vi "data analysis test VI.vi"() -> ()   [LabVIEW 2014]
uses:
  <vilib>/imath/engines/lvmath2/RunTimeEngine/BuiltInFunctions/rand/NIMS_rand(1,I32).vi
  <vilib>/imath/engines/lvmath2/RunTimeEngine/BuiltInFunctions/int16/NIMS_int16(real).vi
  <instcachedir>/0/NIMS_int16(real)_1EFE6F78DFBE4E15B93FF25B3B14BD60.lvgen/NIMS_int16(real)_1EFE6F78DFBE4E15B93FF25B3B14BD60_002.vi
  <vilib>/imath/engines/lvmath2/RunTimeEngine/ErrorHandling/NIMS_Error From Error Code.vi
  <vilib>/imath/engines/lvmath2/RunTimeEngine/BuiltInFunctions/zeros/NIMS_V=zeros(I32,I32).vi
  <vilib>/imath/engines/lvmath2/RunTimeEngine/BuiltInFunctions/int16/NIMS_int16(int).vi
  <instcachedir>/0/NIMS_int16(int)_4445A21B29C14FFE9C78603D13E1117B.lvgen/NIMS_int16(int)_4445A21B29C14FFE9C78603D13E1117B_001.vi
  <vilib>/imathl/engines/lvmath/Functions/Error Handling/Create Error.vi
  <vilib>/imath/engines/lvmath2/RunTimeEngine/RangeToken/NIMS_Range_R2 - Integer.vi
  <instcachedir>/0/NIMS_Range_R2 - Integer_2D1304BAF97744E0A293025746CBADFC.lvgen/NIMS_Range_R2 - Integer_2D1304BAF97744E0A293025746CBADFC_000.vi
  <vilib>/imath/engines/lvmath2/RunTimeEngine/CommandStatement/MC_CommandStatement_break.vi
  <vilib>/imath/engines/lvmath2/RunTimeEngine/IndexRead/NIMS V(S).vi
  <instcachedir>/0/NIMS V(S)_0488751826AF41519A22953C041130DC.lvgen/NIMS V(S)_0488751826AF41519A22953C041130DC_004.vi
  <vilib>/imath/engines/lvmath2/RunTimeEngine/IndexReplace/NIMS V(S)=S.vi
  <instcachedir>/0/NIMS V(S)=S_2D52C4EC15D8415E870AEE69FB516CCA.lvgen/NIMS V(S)=S_2D52C4EC15D8415E870AEE69FB516CCA_003.vi
  <vilib>/imath/engines/lvmath2/RunTimeEngine/ErrorHandling/NIMS_Create Error From Enums.vi
  <instcachedir>/0/NIMS_int16(real)_1EFE6F78DFBE4E15B93FF25B3B14BD60.lvgen/NIMS_int16(real)_1EFE6F78DFBE4E15B93FF25B3B14BD60_000.vi
  <vilib>/imath/engines/lvmath2/RunTimeEngine/NodeEndStatement/NIMS_NodeEndStatement_Output.vi
  <instcachedir>/0/NIMS_NodeEndStatement_Output_53EC0D466D134D7ABD903AC30B43404B.lvgen/NIMS_NodeEndStatement_Output_53EC0D466D134D7ABD903AC30B43404B_012.vi
  <vilib>/imath/engines/lvmath2/RunTimeEngine/ErrorHandling/NIMS_Finalize Error.vi
  <vilib>/imath/engines/lvmath2/RunTimeEngine/BuiltInFunctions/uint16/NIMS_uint16(int).vi
  <instcachedir>/0/NIMS_uint16(int)_AD9B0F7F34DA44259D36ECB142F0DEA3.lvgen/NIMS_uint16(int)_AD9B0F7F34DA44259D36ECB142F0DEA3_001.vi
  <vilib>/imath/engines/lvmath2/RunTimeEngine/IndexReplace/NIMS V(R2)=V.vi
  <instcachedir>/0/NIMS V(R2)=V_680A6DA97A4E4BC09213CA62845C7083.lvgen/NIMS V(R2)=V_680A6DA97A4E4BC09213CA62845C7083_000.vi
  <instcachedir>/0/NIMS_NodeEndStatement_Output_53EC0D466D134D7ABD903AC30B43404B.lvgen/NIMS_NodeEndStatement_Output_53EC0D466D134D7ABD903AC30B43404B_014.vi
panel:
  out "Intensity Graph Y":dbl[][](graph)
  out "Intensity Graph X":dbl[][](graph)
  in  "Scan control":bool
  out "Correlation scanning":bool
  in  "T3 positioning test range (V)":T1
  out "3-1 x correlation":dbl
  out "3-1 y correlation":dbl
  in  "Correlation integration time (s)":dbl
  out "tether forces":waveform(dbl)[](graph)=[{"t0"=timestamp(3.600000000000001 s since 1904-01-01), "dt"=0.1, "Y"=[8.599618085334189, 8.616710768164998], "attributes"=variant("NI_ChannelName"=variant(string "Tether 1"))}, {"t0"=timestamp(3.600000000000001 s since 1904-01-01), "dt"=0.1, "Y"=[8.669934189913317, 8.64500964715035], "attributes"=variant("NI_ChannelName"=variant(string "Tether 2"))}, {"t0"=timestamp(3.600000000000001 s since 1904-01-01), "dt"=0.1, "Y"=[10.029561152841074, 10.043496502647937], "attributes"=variant("NI_ChannelName"=variant(string "Tether 3"))}]
  out "2D tethers":waveform(dbl)[](graph)=[{"t0"=timestamp(3.600000000000001 s since 1904-01-01), "dt"=0.1, "Y"=[930.3826405332136, 929.0101627415797], "attributes"=variant("NI_ChannelName"=variant(string "Tether 1"))}, {"t0"=timestamp(3.600000000000001 s since 1904-01-01), "dt"=0.1, "Y"=[953.5776948104506, 953.7945546499718], "attributes"=variant("NI_ChannelName"=variant(string "Tether 2"))}, {"t0"=timestamp(3.600000000000001 s since 1904-01-01), "dt"=0.1, "Y"=[541.2230047802761, 542.1981030590325], "attributes"=variant("NI_ChannelName"=variant(string "Tether 3"))}]
  in  "Trap 3 Bead Size (nm)":dbl=810.0
  in  "Trap 2 Bead Size (nm)":dbl=810.0
  in  "Trap 1 Bead Size (nm)":dbl=810.0
  out "ratio test":dbl=0.9675233225630537
  in  "Desired forces":T2={"F1x"=7.0, "F1y"=-5.0, "F2x"=-7.0, "F2y"=-5.0}
  in  "Artificial forces":bool=TRUE
  out "Force (pN)":T3={"A_X"=7.0215774989535955, "A_Y"=-4.979745698689579, "B_X"=-7.07501259106649, "B_Y"=-4.989571378686399, "C_X"=-0.031092447141218442, "C_Y"=10.036476588951421}
  out "2D forces":waveform(dbl)[](graph)=[{"t0"=timestamp(3.600000000000001 s since 1904-01-01), "dt"=0.1, "Y"=[7.019682598034811, 7.023472399872379], "attributes"=variant("NI_ChannelName"=variant(string "Trap 1 X"))}, {"t0"=timestamp(3.600000000000001 s since 1904-01-01), "dt"=0.1, "Y"=[-4.967644052914229, -4.991847344464929], "attributes"=variant("NI_ChannelName"=variant(string "Trap 1 Y"))}, {"t0"=timestamp(3.600000000000001 s since 1904-01-01), "dt"=0.1, "Y"=[-7.077163119074762, -7.072862063058218], "attributes"=variant("NI_ChannelName"=variant(string "Trap 2 X"))}, {"t0"=timestamp(3.600000000000001 s since 1904-01-01), "dt"=0.1, "Y"=[-5.008145469476288, -4.97099728789651], "attributes"=variant("NI_ChannelName"=variant(string "Trap 2 Y"))}, {"t0"=timestamp(3.600000000000001 s since 1904-01-01), "dt"=0.1, "Y"=[-0.04011787687321292, -0.022067017409223958], "attributes"=variant("NI_ChannelName"=variant(string "Trap 3 X"))}, {"t0"=timestamp(3.600000000000001 s since 1904-01-01), "dt"=0.1, "Y"=[10.02948091750186, 10.043472260400982], "attributes"=variant("NI_ChannelName"=variant(string "Trap 3 Y"))}]
  in  "Calibration 2":u16(ring)=2 items=["None", "Position", "Force"]
  in  "Calibration":u16(ring)=2 items=["None", "Position", "Force"]
  in  "Displacments":T3={"A_X"=0.0605018, "A_Y"=0.0, "B_X"=0.0507675, "B_Y"=0.0, "C_X"=0.0, "C_Y"=0.0}
  out "Positions \nand displacements":cluster{"X":dbl[], "Y":dbl[]}[](graph)=[{"X"=[3856.9999999999714, 3856.9999999999714], "Y"=[0.0, 0.0]}, {"X"=[6090.0, 6090.0], "Y"=[0.0, 0.0]}, {"X"=[4955.144087038793, 4955.144087038793], "Y"=[-1769.6238715781064, -1769.6238715781064]}, {"X"=[3856.9999999999714, 4191.310570740897, 4191.491059074609], "Y"=[0.0, -233.86603568521076, -235.00547478052496]}, {"X"=[6090.0, 5744.658729782919, 5744.868606554591], "Y"=[0.0, -249.3587186230042, -247.50908725459337]}, {"X"=[4955.144087038793, 4952.707973521867, 4953.804091914954], "Y"=[-1769.6238715781064, -1104.0598883108419, -1103.1314121526243]}, {"X"=[4970.637564152725, 4970.637564152725], "Y"=[-789.6571704971775, -789.6571704971775]}, {"X"=[4952.073488776456, 4952.073488776456], "Y"=[-776.497573056027, -776.497573056027]}, {"X"=[4952.159779557513, 4952.159779557513], "Y"=[-802.6979818639647, -802.6979818639647]}, {"X"=[4958.290277495564, 4958.290277495564], "Y"=[-789.6175751390565, -789.6175751390565]}]
  out "Trap Positions":waveform(dbl)[](graph)=[{"t0"=timestamp(3.600000000000001 s since 1904-01-01), "dt"=0.01, "Y"=[3856.9999999999714, 3856.9999999999714, 3856.9999999999714, 3856.9999999999714, 3856.9999999999714, 3856.9999999999714, 3856.9999999999714, 3856.9999999999714, 3856.9999999999714, 3856.9999999999714, 3856.9999999999714, 3856.9999999999714, 3856.9999999999714, 3856.9999999999714, 3856.9999999999714, 3856.9999999999714, 3856.9999999999714, 3856.9999999999714, 3856.9999999999714, 3856.9999999999714], "attributes"=variant("NI_ChannelName"=variant(string "Trap 1 X"))}, {"t0"=timestamp(3.600000000000001 s since 1904-01-01), "dt"=0.01, "Y"=[6090.0, 6090.0, 6090.0, 6090.0, 6090.0, 6090.0, 6090.0, 6090.0, 6090.0, 6090.0, 6090.0, 6090.0, 6090.0, 6090.0, 6090.0, 6090.0, 6090.0, 6090.0, 6090.0, 6090.0], "attributes"=variant("NI_ChannelName"=variant(string "Trap 2 X"))}, {"t0"=timestamp(3.600000000000001 s since 1904-01-01), "dt"=0.01, "Y"=[4955.144087038793, 4955.144087038793, 4955.144087038793, 4955.144087038793, 4955.144087038793, 4955.144087038793, 4955.144087038793, 4955.144087038793, 4955.144087038793, 4955.144087038793, 4955.144087038793, 4955.144087038793, 4955.144087038793, 4955.144087038793, 4955.144087038793, 4955.144087038793, 4955.144087038793, 4955.144087038793, 4955.144087038793, 4955.144087038793], "attributes"=variant("NI_ChannelName"=variant(string "Trap 3 X"))}, {"t0"=timestamp(3.600000000000001 s since 1904-01-01), "dt"=0.01, "Y"=[-1769.6238715781064, -1769.6238715781064, -1769.6238715781064, -1769.6238715781064, -1769.6238715781064, -1769.6238715781064, -1769.6238715781064, -1769.6238715781064, -1769.6238715781064, -1769.6238715781064, -1769.6238715781064, -1769.6238715781064, -1769.6238715781064, -1769.6238715781064, -1769.6238715781064, -1769.6238715781064, -1769.6238715781064, -1769.6238715781064, -1769.6238715781064, -1769.6238715781064], "attributes"=variant("NI_ChannelName"=variant(string "Trap 3 Y"))}]
  in  "Plot Trap Positions":u16(ring)=1 items=["Relative to Base", "Absolute Positions"]
  in  "Piezo trap y\noffset (V)":dbl=0.6709036530655844
  in  "Piezo trap x\noffset (V)":dbl=-6.361797973205792
  in  "Piezo Trap Y cal (nm/V)":dbl=279.6
  in  "Piezo Trap X cal (nm/V)":dbl=362.7
  in  "AOM X Cal (nm/MHz)":dbl=203.0
  in  "Trap Pos. Disp. Downsample":dbl=1000.0 caption="Trap Downsample"
  in  "Trap 3 Y (V)":dbl=7.0
  in  "Trap 3 X (V)":dbl=7.3
  in  "Trap2 X (MHz)":dbl=90.0
  in  "Trap 1 X (MHz)":dbl=79.0
  in  "Negate Axis":T4={"T1 X"=FALSE, "T2 X"=FALSE, "T3 X"=FALSE, "T3 Y"=TRUE}
  out "Mean":dbl=7.048295045010043 caption="Mean (pN)" format="%#_3g"
  out "T1 X":dbl=7.0215774989535955 caption="T1 X (pN)" format="%0.2f"
  out "T2 X":dbl=7.07501259106649 caption="T2 X (pN)" format="%0.2f"
  out "Difference":dbl=-0.053435092112894544 caption="Difference (pN)" format="%.2g"
  out "Force":waveform(dbl)[](graph)=[{"t0"=timestamp(3.600000000000001 s since 1904-01-01), "dt"=0.1, "Y"=[7.019682598034811, 7.023472399872379], "attributes"=variant("NI_ChannelName"=variant(string "Trap 1 X"))}, {"t0"=timestamp(3.600000000000001 s since 1904-01-01), "dt"=0.1, "Y"=[7.077163119074762, 7.072862063058218], "attributes"=variant("NI_ChannelName"=variant(string "Trap 2 X"))}, {"t0"=timestamp(3.600000000000001 s since 1904-01-01), "dt"=0.1, "Y"=[7.048422858554787, 7.048167231465298], "attributes"=variant("NI_ChannelName"=variant(string "Mean"))}]
  in  "Mean Trap Positions (nm)":T5={"T1 X"=3856.9999999999714, "T2 X"=6090.0, "T3 X"=4955.144087038793, "T3 Y"=-1769.6238715781064} {"T3 Y" format="%#_6f"; "T3 X" format="%#_6f"; "T2 X" format="%#_6f"; "T1 X" format="%#_6f"}
  in  "Path":path=path "C:/Data/180321/current.off"
  in  "Read Cal":bool
  out "Read cal error":errorcluster
  in  "T3 calibration":T6={"alpha_x (nm/V)"=705.7585317734071, "offset_x (mV)"=-72.05792299729328, "kappa_x (pN/nm)"=0.32935966730993543, "alpha_y (nm/V)"=745.2903215958727, "kappa_y (pN/nm)"=0.3013829224432179, "offset_y (mV)"=22.362021368510735} {"offset_y (mV)" format="%#_2g"; "kappa_y (pN/nm)" min=0.0 step=0.001 format="%#_2g"; "alpha_y (nm/V)" step=10.0 format="%#_3g"; "kappa_x (pN/nm)" min=0.0 step=0.001 format="%#_2g"; "offset_x (mV)" format="%#_2g"; "alpha_x (nm/V)" step=10.0 format="%#_3g"}
  in  "T2 calibration":T6={"alpha_x (nm/V)"=564.800175494257, "offset_x (mV)"=-41.69276077209905, "kappa_x (pN/nm)"=0.40986489188657144, "alpha_y (nm/V)"=679.2654766858733, "kappa_y (pN/nm)"=0.40168200230832185, "offset_y (mV)"=-0.41558808755755094} {"offset_y (mV)" format="%#_2g"; "kappa_y (pN/nm)" min=0.0 step=0.001 format="%#_2g"; "alpha_y (nm/V)" step=10.0 format="%#_3g"; "kappa_x (pN/nm)" min=0.0 step=0.001 format="%#_2g"; "offset_x (mV)" format="%#_2g"; "alpha_x (nm/V)" step=10.0 format="%#_3g"}
  in  "T1 calibration":T6={"alpha_x (nm/V)"=544.9680094639928, "offset_x (mV)"=-33.70790453197266, "kappa_x (pN/nm)"=0.4199497839674786, "alpha_y (nm/V)"=662.8467814087468, "kappa_y (pN/nm)"=0.424828174673538, "offset_y (mV)"=32.28801513873096} {"offset_y (mV)" format="%#_2g"; "kappa_y (pN/nm)" min=0.0 step=0.001 format="%#_2g"; "alpha_y (nm/V)" step=10.0 format="%#_3g"; "kappa_x (pN/nm)" min=0.0 step=0.001 format="%#_2g"; "offset_x (mV)" format="%#_2g"; "alpha_x (nm/V)" step=10.0 format="%#_3g"}
  in  "Multi-MCL offset array":T7(array[cluster])
  in  "Two Trap Offset Values":T8={"Trap 1X offset"=array[1799 elements], "Trap 2X offset"=array[1799 elements]}
  in  "MCL offset scanning range (V)":T9={"Min X"=6.0, "Max X"=9.0, "Min Y"=5.0, "Max Y"=8.0, "Scan increment"=1.0}
  in  "Dynamic offset\nupdate":bool=TRUE
  in  "Offset file step size":dbl=0.1
  out "Array":i16[](array[numeric])
  in  "stop":bool
  in  "Multiple-MCL offset?":bool=TRUE
  in  "DMA period (s)":dbl=0.2
  in  "dataperiod (us)":dbl=10.0
  in  "trap sets":u32=2
  in  "Flip X Sign":bool
  in  "Detector Type":string(combo)="IR-QPD + PSD + FB-QPD X position"
  in  "Trap Disp. Downsample":dbl=10000.0 caption="Downsample" max=20000.0
  out "All Signals":waveform(dbl)[](graph)=[{"t0"=timestamp(3.600000000000001 s since 1904-01-01), "dt"=0.1, "Y"=[0.0008898377716559546, 0.000803887358432814], "attributes"=variant("NI_ChannelName"=variant(string "T1 Y"))}, {"t0"=timestamp(3.600000000000001 s since 1904-01-01), "dt"=0.1, "Y"=[-0.004640863177226808, -0.00462430364248546], "attributes"=variant("NI_ChannelName"=variant(string "T1 X"))}, {"t0"=timestamp(3.600000000000001 s since 1904-01-01), "dt"=0.1, "Y"=[0.997039704580851, 0.997039704580851], "attributes"=variant("NI_ChannelName"=variant(string "T1 Sum"))}, {"t0"=timestamp(3.600000000000001 s since 1904-01-01), "dt"=0.1, "Y"=[-0.01875053565962656, -0.018614386287113534], "attributes"=variant("NI_ChannelName"=variant(string "T2 Y"))}, {"t0"=timestamp(3.600000000000001 s since 1904-01-01), "dt"=0.1, "Y"=[-0.07344958677685948, -0.07343100704009785], "attributes"=variant("NI_ChannelName"=variant(string "T2 X"))}, {"t0"=timestamp(3.600000000000001 s since 1904-01-01), "dt"=0.1, "Y"=[0.997039704580851, 0.997039704580851], "attributes"=variant("NI_ChannelName"=variant(string "T2 Sum"))}, {"t0"=timestamp(3.600000000000001 s since 1904-01-01), "dt"=0.1, "Y"=[-2.8313437404346336e-05, -2.907866544230067e-06], "attributes"=variant("NI_ChannelName"=variant(string "T1 FB X"))}, {"t0"=timestamp(3.600000000000001 s since 1904-01-01), "dt"=0.1, "Y"=[0.997039704580851, 0.997039704580851], "attributes"=variant("NI_ChannelName"=variant(string "T1 FB Sum"))}, {"t0"=timestamp(3.600000000000001 s since 1904-01-01), "dt"=0.1, "Y"=[-2.684419957147232e-05, 1.8702173247627797e-05], "attributes"=variant("NI_ChannelName"=variant(string "T2 FB X"))}, {"t0"=timestamp(3.600000000000001 s since 1904-01-01), "dt"=0.1, "Y"=[0.997039704580851, 0.997039704580851], "attributes"=variant("NI_ChannelName"=variant(string "T2 FB Sum"))}, {"t0"=timestamp(3.600000000000001 s since 1904-01-01), "dt"=0.1, "Y"=[0.06976369758187939, 0.06982598714416899], "attributes"=variant("NI_ChannelName"=variant(string "T3 Y/ PSD Y"))}, {"t0"=timestamp(3.600000000000001 s since 1904-01-01), "dt"=0.1, "Y"=[-0.07324104683195597, -0.07316339149066425], "attributes"=variant("NI_ChannelName"=variant(string "T3 X / PSD X"))}, {"t0"=timestamp(3.600000000000001 s since 1904-01-01), "dt"=0.1, "Y"=[0.997039704580851, 0.997039704580851], "attributes"=variant("NI_ChannelName"=variant(string "T3 Sum / PSD sum"))}]
  # "1 D forces traps 1 and 2"
  # "2D forces"
  # "2D tethers"
  # "Individual tether forces"
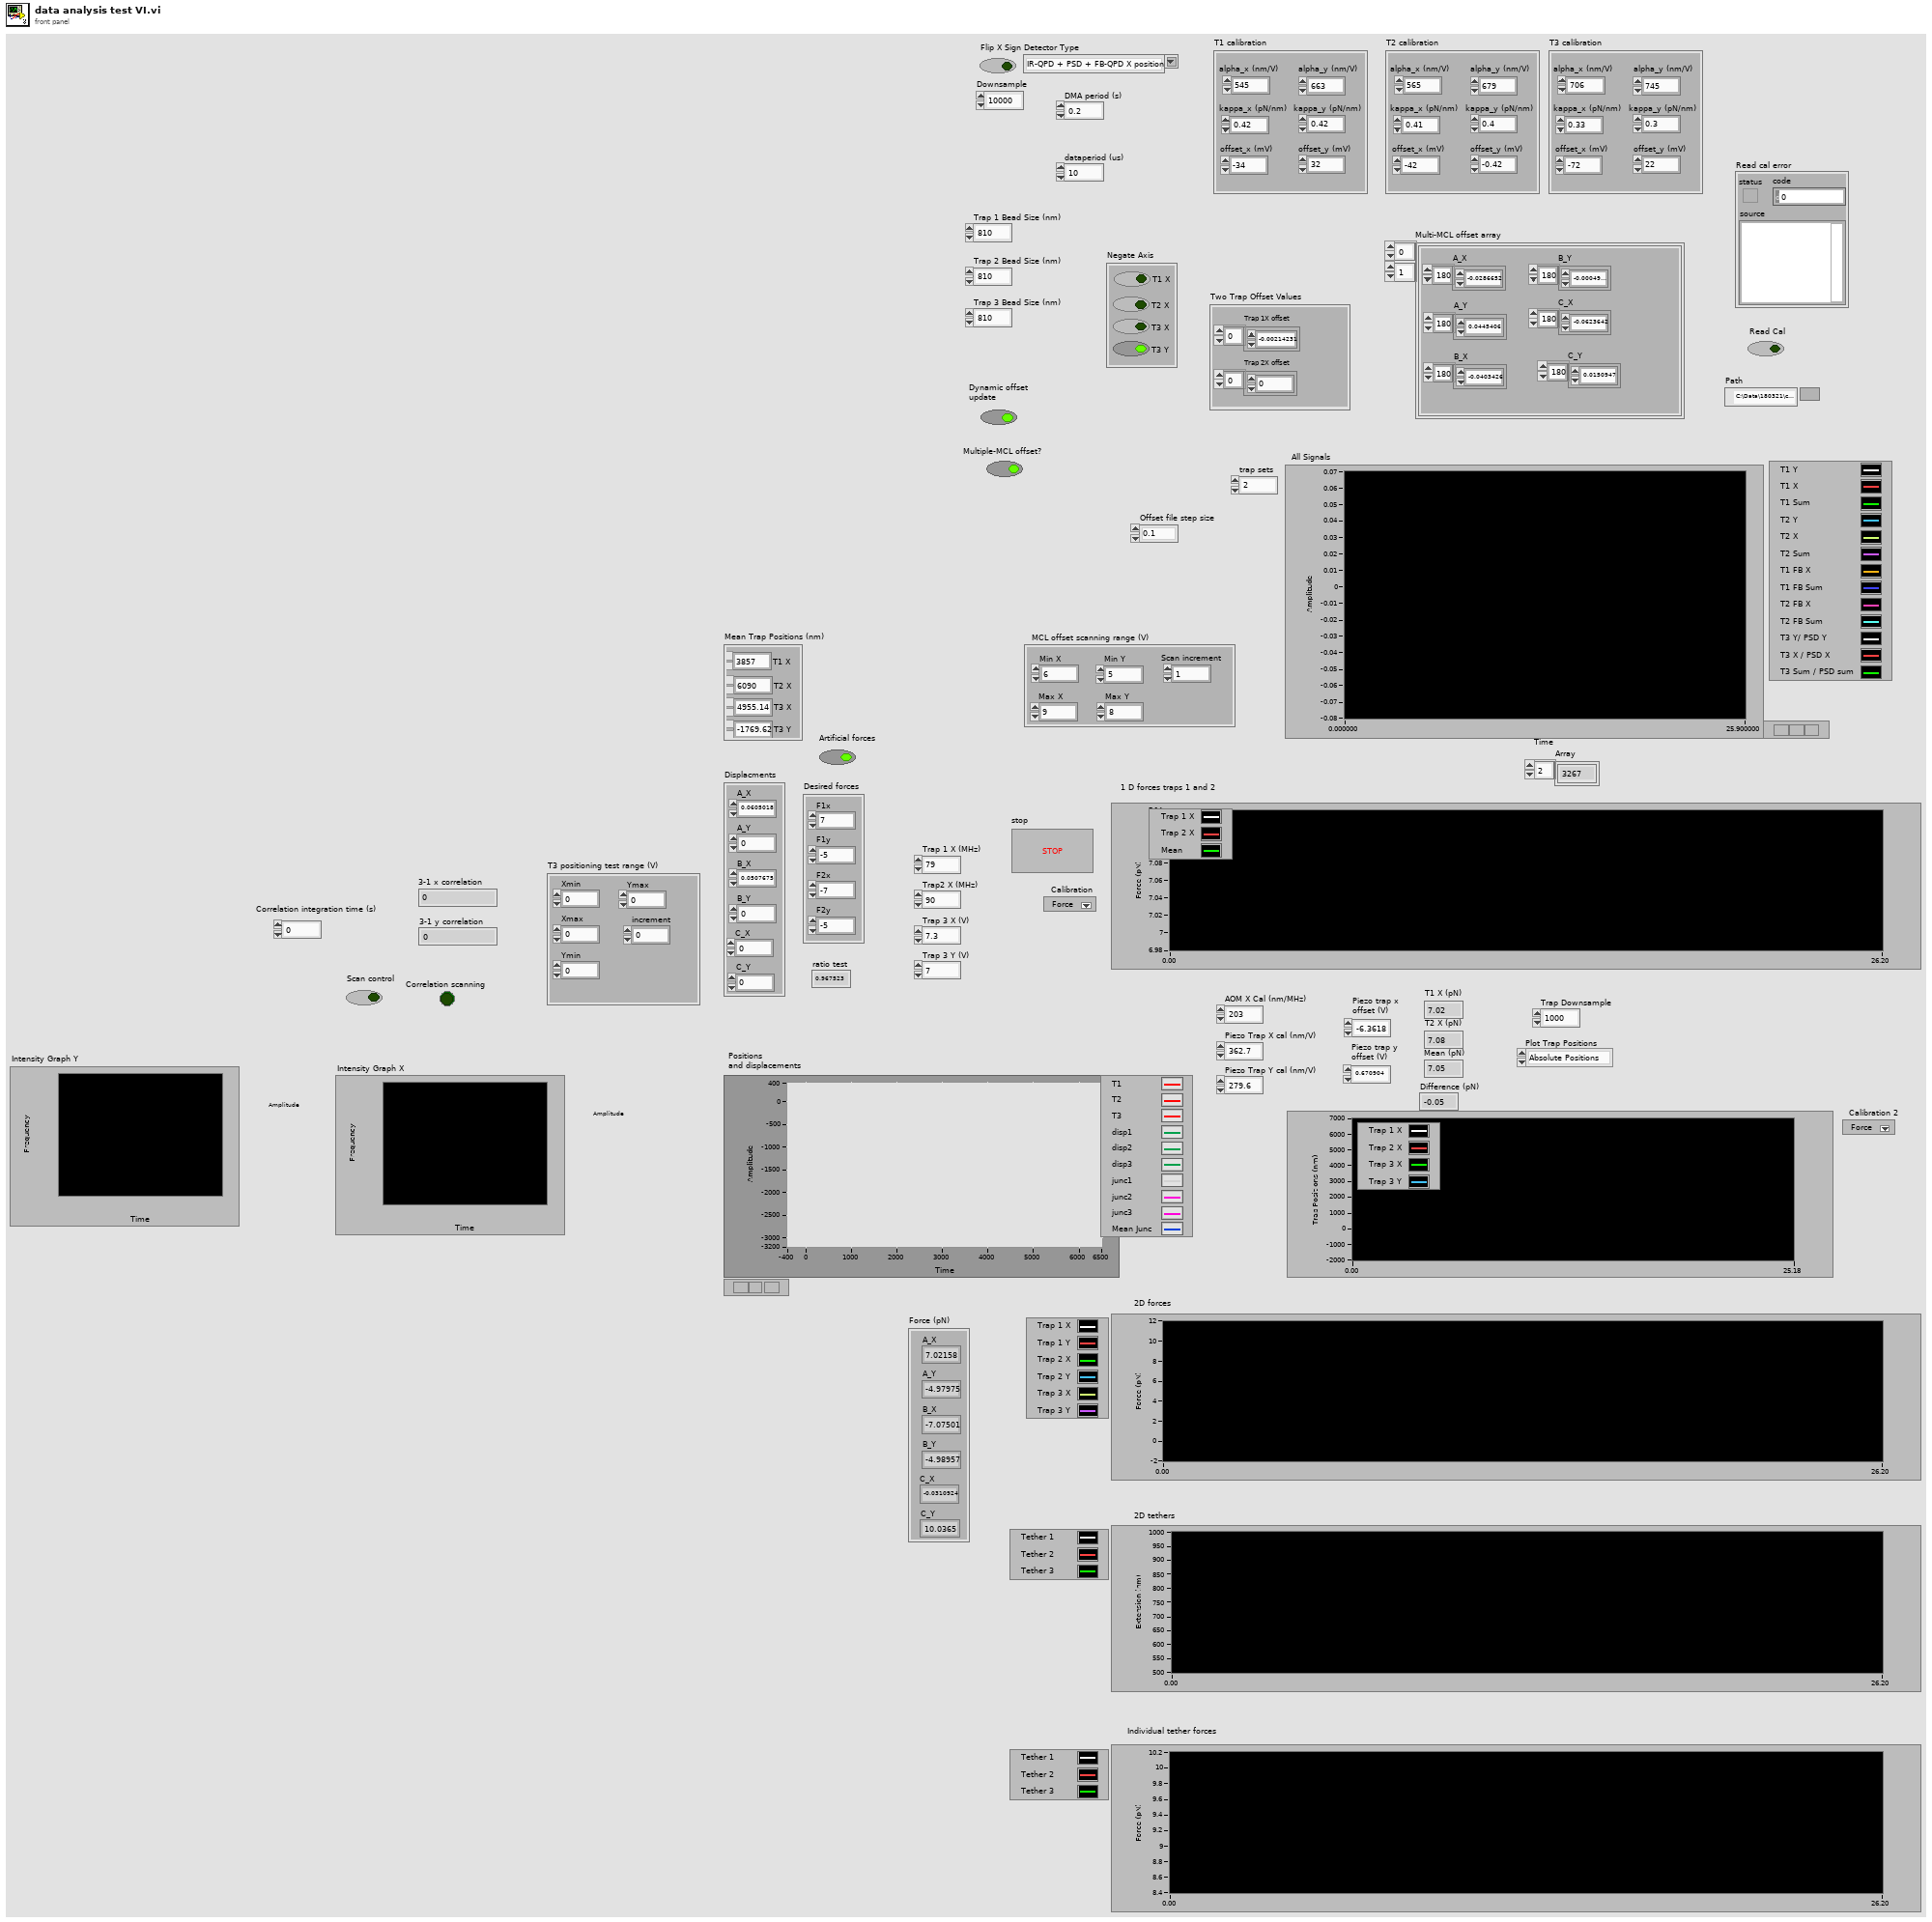
[diagram p1: front panel]
types:
  T1 = cluster{"Xmin":dbl, "Xmax":dbl, "Ymin":dbl, "Ymax":dbl, "increment":dbl}
  T2 = cluster{"F1x":dbl, "F1y":dbl, "F2x":dbl, "F2y":dbl}
  T3 = cluster{"A_X":dbl, "A_Y":dbl, "B_X":dbl, "B_Y":dbl, "C_X":dbl, "C_Y":dbl}
  T4 = cluster{"T1 X":bool, "T2 X":bool, "T3 X":bool, "T3 Y":bool}
  T5 = cluster{"T1 X":dbl, "T2 X":dbl, "T3 X":dbl, "T3 Y":dbl}
  T6 = cluster{"alpha_x (nm/V)":dbl, "offset_x (mV)":dbl, "kappa_x (pN/nm)":dbl, "alpha_y (nm/V)":dbl, "kappa_y (pN/nm)":dbl, "offset_y (mV)":dbl}
  T7 = cluster{"A_X":dbl[], "A_Y":dbl[], "B_X":dbl[], "B_Y":dbl[], "C_X":dbl[], "C_Y":dbl[]}[][]
  T8 = cluster{"Trap 1X offset":dbl[], "Trap 2X offset":dbl[]}
  T9 = cluster{"Min X":dbl, "Max X":dbl, "Min Y":dbl, "Max Y":dbl, "Scan increment":dbl}
  T10 = enum16{"open", "replace", "create", "open or create", "replace or create", "replace or create with confirmation"}
  T11 = enum16{"big-endian, network order", "native, host order", "little-endian"}
  T12 = cluster{"alpha_x (nm/V)":dbl, "offset_x (mV)":dbl, "kappa_x (pN/nm)":dbl, "alpha_y (nm/V)":dbl, "kappa_y (pN/nm)":dbl, "offset_y (mV)":dbl}[]
  T13 = cluster{"[0]":dbl, "[1]":dbl, "[2]":dbl, "[3]":dbl, "[4]":dbl, "[5]":dbl}
  T14 = cluster{"Output trap positions[0]":cluster{"X":dbl[], "Y":dbl[]}, "Output trap positions[1]":cluster{"X":dbl[], "Y":dbl[]}, "Output trap positions[2]":cluster{"X":dbl[], "Y":dbl[]}}
  T15 = cluster{"X correlation":dbl, "Y correlation":dbl}
  T16 = cluster{"T1 X":dbl, "T2 X":dbl, "Mean":dbl, "Difference":dbl}
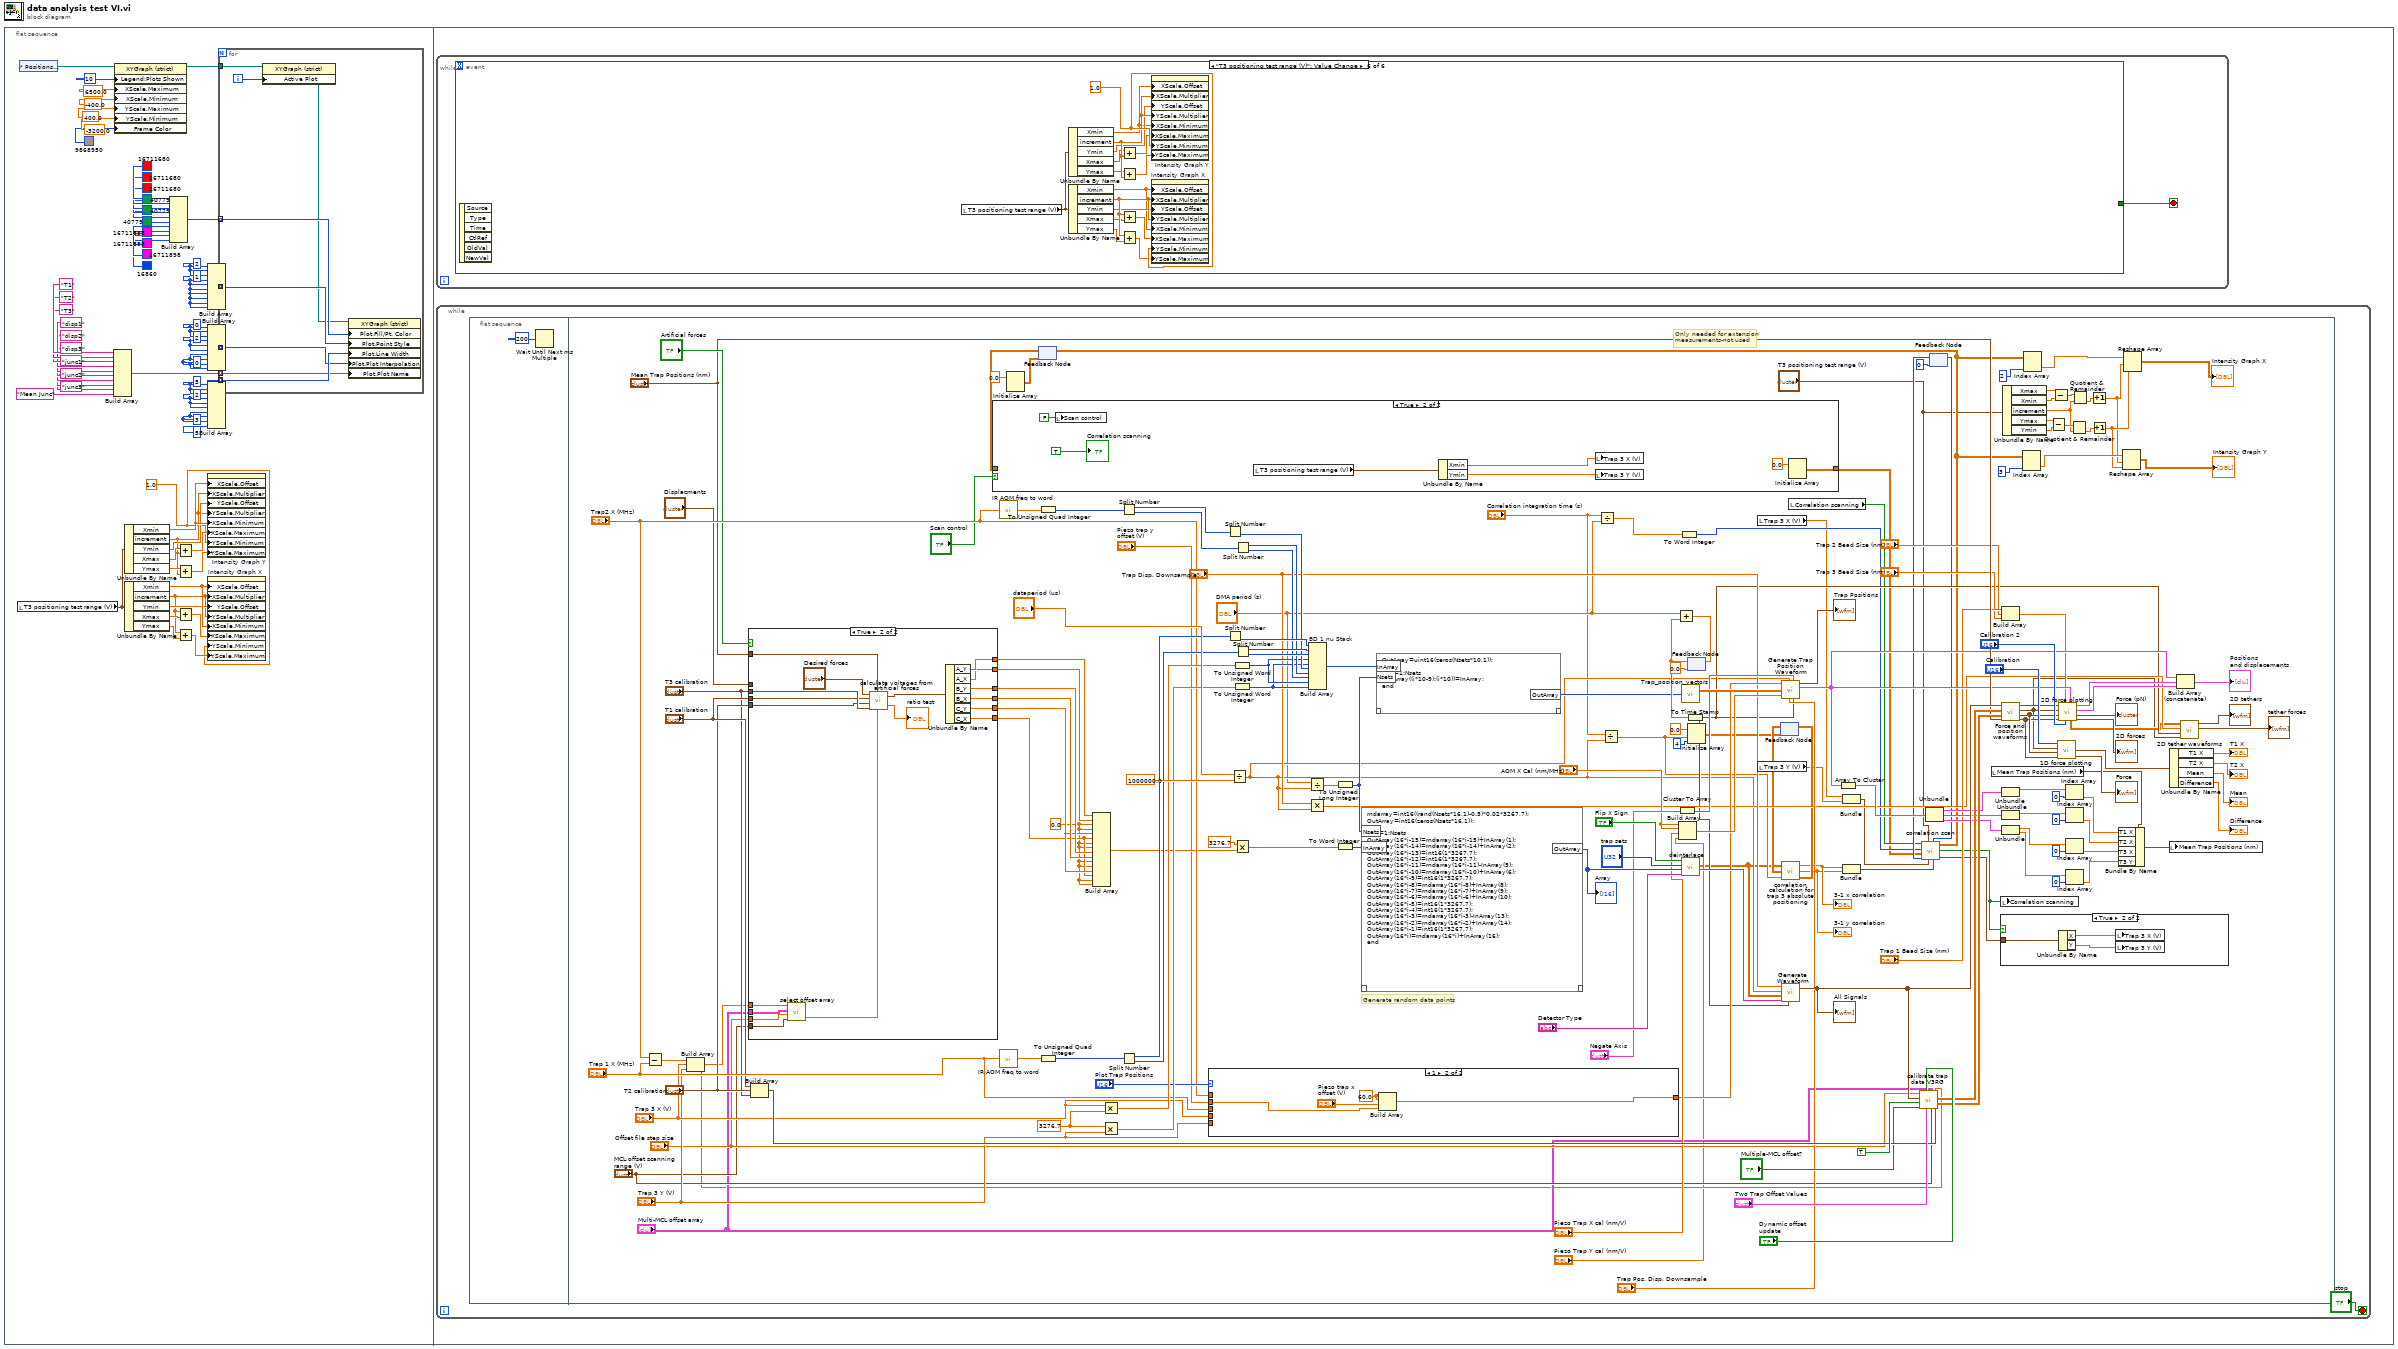
[diagram p0: block diagram]
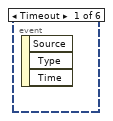
[diagram p2: hidden frame]
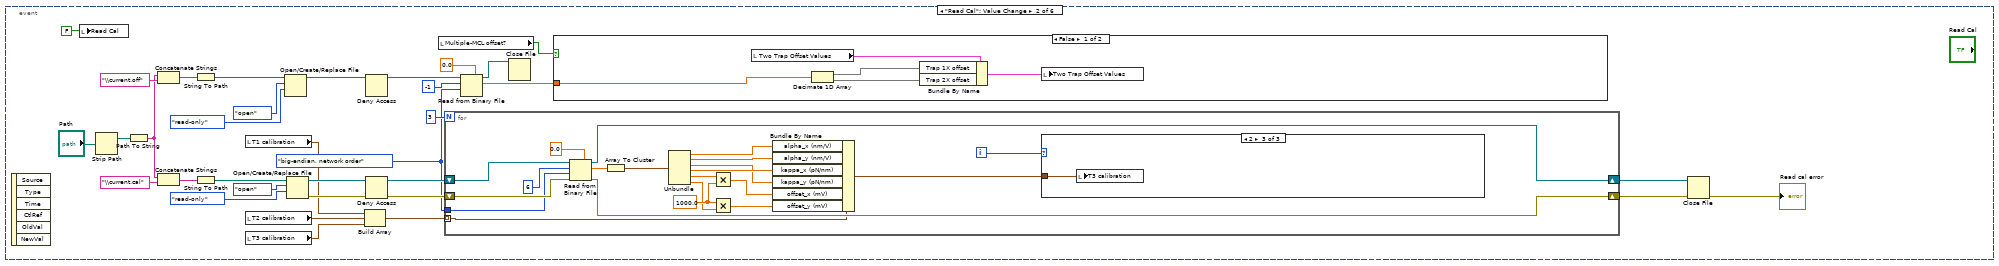
[diagram p3: hidden frame]
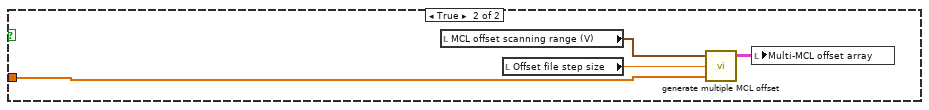
[diagram p4: hidden frame]
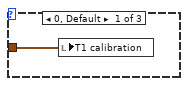
[diagram p5: hidden frame]
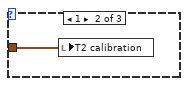
[diagram p6: hidden frame]
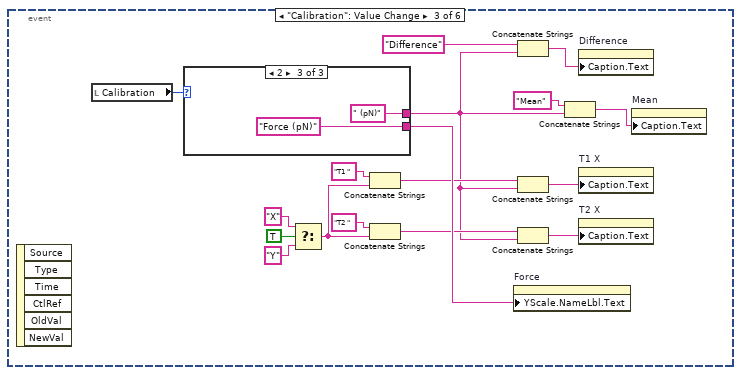
[diagram p7: hidden frame]
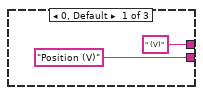
[diagram p8: hidden frame]
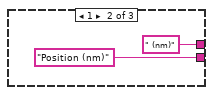
[diagram p9: hidden frame]
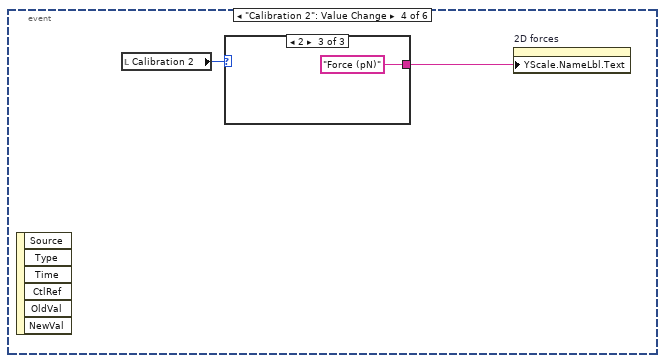
[diagram p10: hidden frame]
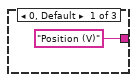
[diagram p11: hidden frame]
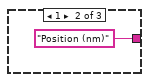
[diagram p12: hidden frame]
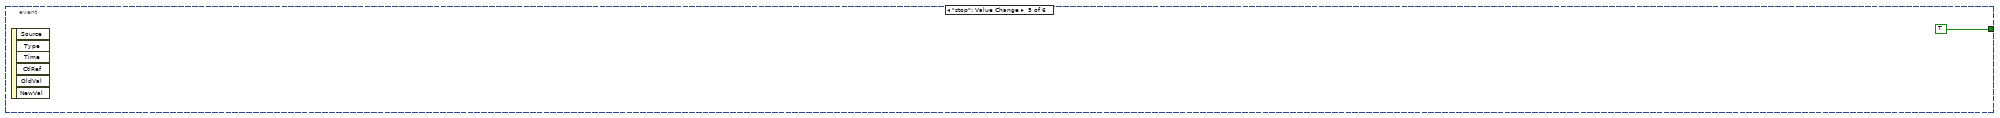
[diagram p13: hidden frame]
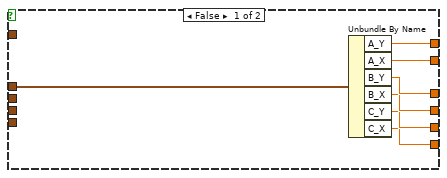
[diagram p16: hidden frame]
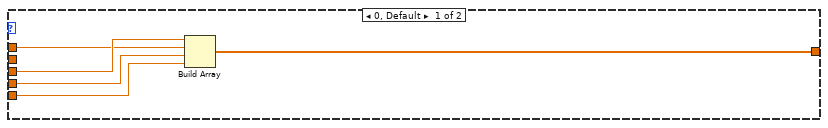
[diagram p17: hidden frame]
diagram:
  n1 = flat-sequence {
    frame #0 {
      w1 = 1.0
      w29 = 0
      w30 = 2
      w31 = 0
      w34 = 3
      w35 = 2
      w36 = 5
      w38 = 1
      w39 = 2
      n2 = local read "T3 positioning test range (V)"() -> (w16:T1)
      n3 = control-ref of="Positions \nand displacements"() -> (w58:refnum<vi>)
      n4 = Build Array("T1", "T2", "T3", "disp1", "disp2", "disp3", "junc1", "junc2", "junc3", "Mean Junc") -> (w17:string[])
      n5 = property class="XYGraph (strict)"(reference=w58, "Legend:Plots Shown"=10, "XScale.Maximum"=6500.0, "XScale.Minimum"=-400.0, "YScale.Maximum"=400.0, "YScale.Minimum"=-3200.0, "Frame Color"=u32 9868950) -> (reference out=w51:refnum<vi>)  [unwired: 1 in, 1 out]
      n6 = Unbundle By Name(w16) -> ("Xmin"=w15:dbl, "increment"=w10:dbl, "Ymin"=w12:dbl, "Xmax"=w14:dbl, "Ymax"=w11:dbl)
      n7 = Unbundle By Name(w16) -> ("Xmin"=w8:dbl, "increment"=w3:dbl, "Ymin"=w7:dbl, "Xmax"=w6:dbl, "Ymax"=w4:dbl)
      n8 = Build Array(u32 16711680, u32 16711680, u32 16711680, u32 40779, u32 40779, u32 40779, u32 16711898, u32 16711898, u32 16711898, u32 16860) -> (w40:u32[])
      n9 = Add(x=w14, y=w10) -> (x+y=w13:dbl)
      n10 = Add(x=w11, y=w10) -> (x+y=w9:dbl)
      n11 = Add(x=w3, y=w6) -> (x+y=w5:dbl)
      n12 = Add(x=w3, y=w4) -> (x+y=w2:dbl)
      n13 = Build Array(w39, w39, w39, w38, w38, w38, w38, w38, w38, w38) -> (w37:i32[])
      n14 = Build Array(w31, w31, w31, w30, w30, w30, w29, w29, w29, w29) -> (w28:i32[])
      n15 = Build Array(w36, w36, w36, w35, w35, w35, w34, w34, w34, 5) -> (w32:i32[])
      n16 = property on="Intensity Graph Y" class="IntGraph (strict)"("XScale.Offset"=w15, "XScale.Multiplier"=w10, "YScale.Offset"=w12, "YScale.Multiplier"=w10, "XScale.Minimum"=w15, "XScale.Maximum"=w13, "YScale.Minimum"=w1, "YScale.Maximum"=w9) -> ()  [unwired: 2 in, 2 out]
      n17 = property on="Intensity Graph X" class="IntGraph (strict)"("XScale.Offset"=w8, "XScale.Multiplier"=w3, "YScale.Offset"=w7, "YScale.Multiplier"=w3, "XScale.Minimum"=w8, "XScale.Maximum"=w5, "YScale.Minimum"=w1, "YScale.Maximum"=w2) -> ()  [unwired: 2 in, 2 out]
      n18 = for {
        tunnel: w51 -> [w66]
        tunnel: w40 -> [w64] mode=indexing
        tunnel: w37 -> [w63] mode=indexing
        tunnel: w32 -> [w62] mode=indexing
        tunnel: w28 -> [w61] mode=indexing
        tunnel: w17 -> [w59] mode=indexing
        i -> [w65]
        n19 = property class="XYGraph (strict)"(reference=w66, "Active Plot"=w65) -> (reference out=w60:refnum<vi>)  [unwired: 1 in, 1 out]
        n20 = property class="XYGraph (strict)"(reference=w60, "Plot.Fill/Pt. Color"=w64, "Plot.Point Style"=w63, "Plot.Line Width"=w62, "Plot.Plot Interpolation"=w61, "Plot.Plot Name"=w59) -> ()  [unwired: 1 in, 2 out]
      }
    }
    frame #1 {
      n21 = while {
        stop <- w67 stop-if-true
        n22 = event shown="[5] \"T3 positioning test range (V)\": Value Change" {
          selector: _ -> [_ _ _ _ _ _]
          dyn-events: _ -> [_ _ _ _ _ _]
          timeout: _ -> [_ _ _ _ _ _]
          tunnel: [_ _ _ _ TRUE _] -> w67
          event Timeout {
            n23 = event-data() -> ()  [unwired: 1 in, 3 out]
          }
          event "Read Cal": Value Change {
            w79 = T11."big-endian, network order" ("byte order (0:big-endian, network order)")
            n24 = event-data() -> ()  [unwired: 1 in, 6 out]
            n25 = local write "Read Cal"(FALSE) -> ()
            n26 = Strip Path(path="Path") -> (stripped path=w88:path)  [unwired: 1 out]
            n27 = Path To String(path=w88) -> (string=w93:string)
            n28 = Concatenate Strings(w93, "\\current.off" ("string")) -> (w95:string)
            n29 = Concatenate Strings(w93, "\\current.cal" ("string")) -> (w90:string)
            n30 = String To Path(string=w95) -> (path=w98:path)
            n31 = String To Path(string=w90) -> (path=w91:path)
            n32 = local read "T1 calibration"() -> (w78:T6)
            n33 = local read "T2 calibration"() -> (w77:T6)
            n34 = local read "T3 calibration"() -> (w76:T6)
            n35 = Open/Create/Replace File(file path (use dialog)=w98, operation (0:open)=T10."open", access (0:read/write)=enum16{"read/write", "read-only", "write-only"}."read-only") -> (refnum out=w99:refnum<file>)  [unwired: 1 in, 4 out]
            n36 = Open/Create/Replace File(file path (use dialog)=w91, operation (0:open)=T10."open", access (0:read/write)=enum16{"read/write", "read-only", "write-only"}."read-only") -> (refnum out=w85:refnum<file>, error out=w92:errorcluster)  [unwired: 1 in, 3 out]
            n37 = Build Array(w78, w77, w76) -> (w75:T12)
            n38 = Deny Access(7:w99) -> (3:w100:refnum<file>)  [unwired: 1 in, 2 out]
            n39 = Deny Access(4:w92, 7:w85) -> (0:w80:errorcluster, 3:w81:refnum<file>)  [unwired: 1 out]
            n40 = local read "Multiple-MCL offset?"() -> (w73:bool)
            n41 = for {
              N: 3 -> [_]
              shift-right: [w117] -> w70
              shift-left: w81 -> [w118]
              shift-right: [w115] -> w69
              shift-left: w80 -> [w116]
              tunnel: w79 -> [w114]
              tunnel: w75 -> [w113] mode=indexing
              i -> [w112]
              w130 = 1000.0
              n42 = Read from Binary File(5:0.0, 8:w116, 9:w114, 10:6 ("count (1)"), 11:w118) -> (0:w115:errorcluster, 2:w119:dbl[], 3:w117:refnum<file>)  [unwired: 2 out]
              n43 = Array To Cluster(array=w119) -> (cluster=w122:T13)
              n44 = Unbundle(w122) -> ("[0]"=w123:dbl, "[1]"=w124:dbl, "[2]"=w128:dbl, "[3]"=w125:dbl, "[4]"=w129:dbl, "[5]"=w126:dbl)
              n45 = Multiply(x=w129, y=w130) -> (x*y=w131:dbl)
              n46 = Multiply(x=w130, y=w126) -> (x*y=w127:dbl)
              n47 = Bundle By Name(cluster=w113, "alpha_x (nm/V)"=w123, "alpha_y (nm/V)"=w124, "kappa_x (pN/nm)"=w128, "kappa_y (pN/nm)"=w125, "offset_x (mV)"=w131, "offset_y (mV)"=w127) -> (w111:T6)
              n48 = case shown="2" w112 {
                tunnel: w111 -> [w132 w133 w134]
                frame 0, Default {
                  n49 = local write "T1 calibration"(w132) -> ()
                }
                frame 1 {
                  n50 = local write "T2 calibration"(w133) -> ()
                }
                frame 2 {
                  n51 = local write "T3 calibration"(w134) -> ()
                }
              }
            }
            n52 = Read from Binary File(5:0.0, 9:w79, 10:-1 ("count (1)"), 11:w100) -> (2:w72:dbl[], 3:w83:refnum<file>)  [unwired: 1 in, 3 out]
            n53 = Close File(refnum=w83) -> ()  [unwired: 1 in, 2 out]
            n54 = case shown="False" w73 {
              tunnel: w72 -> [w106 w108]
              frame False {
                n55 = local read "Two Trap Offset Values"() -> (w105:T8)
                n56 = Decimate 1D Array(w106) -> (w104:dbl[], w103:dbl[])
                n57 = Bundle By Name(cluster=w105, "Trap 1X offset"=w104, "Trap 2X offset"=w103) -> (w102:T8)
                n58 = local write "Two Trap Offset Values"(w102) -> ()
              }
              frame True {
                n59 = local read "MCL offset scanning range (V)"() -> (w110:T9)
                n60 = local read "Offset file step size"() -> (w109:dbl)
                n61 = call "generate multiple MCL offset.vi"("Offset array"=w108, "offset file step size"=w109, "MCL offset scanning range (V)"=w110) -> ("Output array"=w107:T7)  [unwired: 2 out]
                n62 = local write "Multi-MCL offset array"(w107) -> ()
              }
            }
            n63 = Close File(refnum=w70, error in=w69) -> (error out=→"Read cal error":errorcluster)  [unwired: 1 out]
          }
          event "Calibration": Value Change {
            n64 = event-data() -> ()  [unwired: 1 in, 6 out]
            n65 = local read "Calibration"() -> (w151:u16)
            n66 = case shown="2" w151 {
              tunnel: ["Position (V)" ("Label.Text") "Position (nm)" ("Label.Text") "Force (pN)" ("Label.Text")] -> w150
              tunnel: [" (V)" ("Label.Text") " (nm)" ("Label.Text") " (pN)" ("Label.Text")] -> w139
              frame 0, Default {
              }
              frame 1 {
              }
              frame 2 {
              }
            }
            n67 = Select(t="X" ("Label.Text"), s=TRUE, f="Y" ("Label.Text")) -> (s? t:f=w144:string)
            n68 = Concatenate Strings("T1 " ("Label.Text"), w144) -> (w147:string)
            n69 = Concatenate Strings("T2 " ("Label.Text"), w144) -> (w148:string)
            n70 = property on="Force" class="WFChart (strict)"("YScale.NameLbl.Text"=w150) -> ()  [unwired: 2 in, 2 out]
            n71 = Concatenate Strings("Difference" ("Label.Text"), w139) -> (w135:string)
            n72 = Concatenate Strings(w147, w139) -> (w137:string)
            n73 = Concatenate Strings(w148, w139) -> (w136:string)
            n74 = Concatenate Strings("Mean" ("Label.Text"), w139) -> (w138:string)
            n75 = property on="Difference" class="DigNum (strict)"("Caption.Text"=w135) -> ()  [unwired: 2 in, 2 out]
            n76 = property on="T1 X" class="DigNum (strict)"("Caption.Text"=w137) -> ()  [unwired: 2 in, 2 out]
            n77 = property on="T2 X" class="DigNum (strict)"("Caption.Text"=w136) -> ()  [unwired: 2 in, 2 out]
            n78 = property on="Mean" class="DigNum (strict)"("Caption.Text"=w138) -> ()  [unwired: 2 in, 2 out]
          }
          event "Calibration 2": Value Change {
            n79 = event-data() -> ()  [unwired: 1 in, 6 out]
            n80 = local read "Calibration 2"() -> (w159:u16)
            n81 = case shown="2" w159 {
              tunnel: ["Position (V)" ("Label.Text") "Position (nm)" ("Label.Text") "Force (pN)" ("Label.Text")] -> w158
              frame 0, Default {
              }
              frame 1 {
              }
              frame 2 {
              }
            }
            n82 = property on="2D forces" class="WFChart (strict)"("YScale.NameLbl.Text"=w158) -> ()  [unwired: 2 in, 2 out]
          }
          event "stop": Value Change {
            n83 = event-data() -> ()  [unwired: 1 in, 6 out]
          }
          event "T3 positioning test range (V)": Value Change {
            w179 = 1.0
            n84 = event-data() -> ()  [unwired: 1 in, 6 out]
            n85 = local read "T3 positioning test range (V)"() -> (w164:T1)
            n86 = Unbundle By Name(w164) -> ("Xmin"=w165:dbl, "increment"=w170:dbl, "Ymin"=w168:dbl, "Xmax"=w166:dbl, "Ymax"=w169:dbl)
            n87 = Unbundle By Name(w164) -> ("Xmin"=w172:dbl, "increment"=w177:dbl, "Ymin"=w173:dbl, "Xmax"=w174:dbl, "Ymax"=w176:dbl)
            n88 = Add(x=w166, y=w170) -> (x+y=w167:dbl)
            n89 = Add(x=w169, y=w170) -> (x+y=w171:dbl)
            n90 = Add(x=w177, y=w174) -> (x+y=w175:dbl)
            n91 = Add(x=w177, y=w176) -> (x+y=w178:dbl)
            n92 = property on="Intensity Graph Y" class="IntGraph (strict)"("XScale.Offset"=w165, "XScale.Multiplier"=w170, "YScale.Offset"=w168, "YScale.Multiplier"=w170, "XScale.Minimum"=w165, "XScale.Maximum"=w167, "YScale.Minimum"=w179, "YScale.Maximum"=w171) -> ()  [unwired: 2 in, 2 out]
            n93 = property on="Intensity Graph X" class="IntGraph (strict)"("XScale.Offset"=w172, "XScale.Multiplier"=w177, "YScale.Offset"=w173, "YScale.Multiplier"=w177, "XScale.Minimum"=w172, "XScale.Maximum"=w175, "YScale.Minimum"=w179, "YScale.Maximum"=w178) -> ()  [unwired: 2 in, 2 out]
          }
        }
      }
      n94 = while {
        stop <- "stop" stop-if-true
        n95 = flat-sequence {
          frame #0 {
            n96 = Wait Until Next ms Multiple(millisecond multiple=u32 200) -> ()  [unwired: 1 out]
          }
          frame #1 {
            w286 = 0.0
            w313 = 3276.7
            # "Only needed for extension\nmeasurements-not used"
            # "Generate random data points"
            n97 = Subtract(x="Trap2 X (MHz)", y="Trap 1 X (MHz)") -> (x-y=w296:dbl)
            n98 = Build Array(w296, "Trap 3 X (V)", "Trap 3 Y (V)") -> (w265:dbl[])
            n99 = case shown="True" "Artificial forces" {
              tunnel: "Displacments" -> [w372 _]
              tunnel: [w371 w388] -> w292
              tunnel: [w370 w387] -> w291
              tunnel: [w369 w386] -> w290
              tunnel: [w368 w384] -> w289
              tunnel: [w367 w383] -> w288
              tunnel: [w366 w385] -> w287
              tunnel: "T1 calibration" -> [_ w381]
              tunnel: "T2 calibration" -> [_ w380]
              tunnel: "T3 calibration" -> [_ w382]
              tunnel: "Mean Trap Positions (nm)" -> [_ w374]
              tunnel: "Offset file step size" -> [_ w379]
              tunnel: "MCL offset scanning range (V)" -> [_ w378]
              tunnel: "Multi-MCL offset array" -> [_ w377]
              tunnel: w265 -> [_ w376]
              frame False {
                n100 = Unbundle By Name(w372) -> ("A_Y"=w371:dbl, "A_X"=w370:dbl, "B_Y"=w369:dbl, "B_X"=w368:dbl, "C_Y"=w367:dbl, "C_X"=w366:dbl)
              }
              frame True {
                n101 = call "select offset array.vi"("MCL offset scanning range (V)"=w378, "Offset File step size"=w379, "Multi-MCL offset array"=w377, "Trap position array"=w376) -> ("Out offsets"=w375:dbl[])  [unwired: 1 out]
                n102 = call "calculate voltages from artificial forces.vi"("offsets"=w375, "Mean Trap Positions (nm)"=w374, "T3 calibration"=w382, "T2 calibration"=w380, "T1 calibration"=w381, "Desired forces (pN)"="Desired forces") -> ("ratio"=→"ratio test":dbl, "Output displacements"=w389:T3)
                n103 = Unbundle By Name(w389) -> ("A_Y"=w388:dbl, "A_X"=w387:dbl, "B_Y"=w386:dbl, "B_X"=w384:dbl, "C_Y"=w383:dbl, "C_X"=w385:dbl)
              }
            }
            n104 = Build Array("T1 calibration", "T2 calibration", "T3 calibration") -> (w341:T12)
            n105 = call "IR AOM freq to word.vi"("Frequency In (MHz)"="Trap2 X (MHz)") -> ("Frequency Word Out (double)"=w299:dbl)
            n106 = call "IR AOM freq to word.vi"("Frequency In (MHz)"="Trap 1 X (MHz)") -> ("Frequency Word Out (double)"=w328:dbl)
            n107 = Initialize Array(0.0) -> (w204:dbl[][])  [unwired: 2 in]
            n108 = feedback #1(w204) -> (w202:dbl[][])
            n109 = case shown="True" "Scan control" {
              tunnel: [w355 w356] -> w201
              tunnel: w202 -> [w355 _]
              frame False {
              }
              frame True {
                n110 = local write "Scan control"(FALSE) -> ()
                n111 = local read "T3 positioning test range (V)"() -> (w359:T1)
                n112 = Unbundle By Name(w359) -> ("Xmin"=w360:dbl, "Ymin"=w361:dbl)
                n113 = local write "Trap 3 X (V)"(w360) -> ()
                n114 = local write "Trap 3 Y (V)"(w361) -> ()
                n115 = Initialize Array(0.0) -> (w356:dbl[][])  [unwired: 2 in]
                "Correlation scanning" <- TRUE
              }
            }
            n116 = To Unsigned Quad Integer(1:w299) -> (0:w321:u64)
            n117 = To Unsigned Quad Integer(1:w328) -> (0:w322:u64)
            n118 = Build Array(w292, w291, w286, w286, w288, w287, w286, w286, w290, w289, w286, w286, w288, w287, w286, w286) -> (w284:dbl[])
            n119 = Multiply(x="Trap 3 X (V)", y=w313) -> (x*y=w315:dbl)
            n120 = Multiply(x=w313, y="Trap 3 Y (V)") -> (x*y=w312:dbl)
            n121 = Split Number(x=w321) -> (hi(x)=w319:u32, lo(x)=w320:u32)
            n122 = Split Number(x=w322) -> (hi(x)=w327:u32, lo(x)=w326:u32)
            n123 = case shown="1" "Plot Trap Positions" {
              tunnel: "Trap 1 X (MHz)" -> [w395 _]
              tunnel: "Trap2 X (MHz)" -> [w394 _]
              tunnel: "Trap 3 X (V)" -> [w393 _]
              tunnel: "Trap 3 Y (V)" -> [w392 _]
              tunnel: [w391 w397] -> w301
              tunnel: "Piezo trap y\noffset (V)" -> [_ w396]
              frame 0, Default {
                n124 = Build Array(w395, w394, w393, w392) -> (w391:dbl[])
              }
              frame 1 {
                w399 = 60.0
                n125 = Build Array(w399, w399, "Piezo trap x\noffset (V)", w396) -> (w397:dbl[])
              }
            }
            n126 = Split Number(x=w319) -> (lo(x)=w318:u16)  [unwired: 1 out]
            n127 = Split Number(x=w327) -> (lo(x)=w325:u16)  [unwired: 1 out]
            n128 = Divide(x="dataperiod (us)", y=1000000.0) -> (x/y=w223:dbl)
            n129 = To Unsigned Word Integer(number=w315) -> (unsigned 16bit integer=w314:u16)
            n130 = To Unsigned Word Integer(number=w312) -> (unsigned 16bit integer=w311:u16)
            n131 = Multiply(x=3276.7, y=w284) -> (x*y=w283:dbl[])
            n132 = Split Number(x=w320) -> (hi(x)=w317:u16, lo(x)=w316:u16)
            n133 = Split Number(x=w326) -> (hi(x)=w324:u16, lo(x)=w323:u16)
            n134 = Build Array "BD 1 nu Stack"(w325, w324, w323, w314, w311, w318, w317, w316, w314, w311) -> (w310:u16[])
            n135 = Divide(x="DMA period (s)", y=w223) -> (x/y=w348:dbl)
            n136 = Multiply(x="Trap Disp. Downsample", y=w223) -> (x*y=w235:dbl)
            n137 = To Unsigned Long Integer(number=w348) -> (unsigned 32bit integer=w282:u32)
            n138 = To Word Integer(number=w283) -> (16bit integer=w281:i16[])
            n139 = mathscript code="rndarray=int16((rand(Nsets*16,1)-0.5)*0.02*3267.7);\nOutArray=int16(zeros(Nsets*16,1));\n\nfor i=1:Nsets\nOutArray(16*i-15)=rndarray(16*i-15)+InArray(1);\nOutArray(16*i-14)=rndarray(16*i-14)+InArray(2);\nOutArray(16*i-13)=int16(1*3267.7);\nOutArray(16*i-12)=int16(1*3267.7);\nOutArray(16*i-11)=rndarray(16*i-11)-InArray(5);\nOutArray(16*i-10)=rndarray(16*i-10)+InArray(6);\nOutArray(16*i-9)=int16(1*3267.7);\nOutArray(16*i-8)=rndarray(16*i-8)+InArray(8);\nOutArray(16*i-7)=rndarray(16*i-7)+InArray(9);\nOutArray(16*i-6)=rndarray(16*i-6)+InArray(10);\nOutArray(16*i-5)=int16(1*3267.7);\nOutArray(16*i-4)=int16(1*3267.7);\nOutArray(16*i-3)=rndarray(16*i-3)-InArray(13);\nOutArray(16*i-2)=rndarray(16*i-2)+InArray(14);\nOutArray(16*i-1)=int16(1*3267.7);\nOutArray(16*i)=rndarray(16*i)+InArray(16);\nend"("Nsets"=w282, "InArray"=w281) -> ("OutArray"=w346:i16[])  [unwired: 1 in, 1 out]
            "Array" <- w346
            n140 = mathscript code="OutArray=uint16(zeros(Nsets*10,1));\n\nfor i=1:Nsets\nOutArray((i*10-9):(i*10))=InArray;\nend"("Nsets"=w282, "InArray"=w310) -> ("OutArray"=w309:u16[])  [unwired: 1 in, 1 out]
            n141 = Divide(x="Correlation integration time (s)", y="DMA period (s)") -> (x/y=w216:dbl)
            n142 = Divide(x="Correlation integration time (s)", y=w223) -> (x/y=w229:dbl)
            n143 = Cluster To Array(cluster="Negate Axis") -> (array=w306:bool[])
            n144 = Build Array("AOM X Cal (nm/MHz)", "AOM X Cal (nm/MHz)", "Piezo Trap X cal (nm/V)", "Piezo Trap Y cal (nm/V)") -> (w303:dbl[])
            n145 = To Word Integer(number=w216) -> (16bit integer=w215:i16)
            n146 = call "Trap_position_vectors.vi"("Data array"=w309) -> ("Output data for plotting"=w308:dbl[][])  [unwired: 1 out]
            n147 = call "deinterlace.vi"("Detector type"="Detector Type", "Data"=w346, "Trap sets"="trap sets", "Flip x sign"="Flip X Sign") -> ("Channel names"=w351:string[], "Deinterlaced normalized data"=w222:dbl[][])  [unwired: 2 out]
            n148 = feedback #2(0.0) -> (w352:dbl)
            n149 = Add(x="DMA period (s)", y=w352) -> (x+y=w353:dbl)
            n150 = To Time Stamp(1:w352) -> (0:w234:timestamp)
            n151 = feedback-in #2(w353) -> ()
            n152 = Initialize Array(0.0, w229, 4) -> (w226:dbl[][])
            n153 = local read "Trap 3 X (V)"() -> (w209:dbl)
            n154 = local read "Trap 3 Y (V)"() -> (w208:dbl)
            n155 = feedback #3(w226) -> (w227:dbl[][])
            n156 = call "Generate Waveform.vi"("Downsampling"="Trap Disp. Downsample", "Data Period (s)"=w223, "Data"=w222, "Plot names"=w351, "Time Stamp"=w234) -> ("Downsampled data"=w337:waveform(dbl)[])  [unwired: 1 out]
            "All Signals" <- w337
            n157 = call "Generate Trap Positiion Waveform.vi"("Base trap positions"=w301, "Data Period (s)"=w223, "Input data"=w308, "Position calibration values"=w303, "Trap Pos. Disp. Downsample (s)"="Trap Pos. Disp. Downsample", "Negate axis"=w306, "Time Stamp"=w234) -> ("Output waveforms"=→"Trap Positions":waveform(dbl)[], "Output trap positions"=w264:cluster{"X":dbl[], "Y":dbl[]}[])  [unwired: 2 in]
            n158 = call "correlation calculation for trap 3 absolute positioning.vi"("Number of sets to average"=w229, "Accumulated array"=w227, "raw data"=w222) -> ("Accumulated array out"=w228:dbl[][], "Y correlation"=w211:dbl, "X correlation"=w212:dbl)
            "3-1 y correlation" <- w211
            "3-1 x correlation" <- w212
            n159 = feedback-in #3(w228) -> ()
            n160 = local read "Correlation scanning"() -> (w214:bool)
            n161 = Array To Cluster(array=w264) -> (cluster=w263:T14)
            n162 = Bundle("Trap 3 X (V)"=w209, "Trap 3 Y (V)"=w208) -> (w207:cluster{"Trap 3 X (V) ":dbl, "Trap 3 Y (V)":dbl})  [unwired: 1 in]
            n163 = Bundle("X correlation"=w212, "Y correlation"=w211) -> (w210:T15)  [unwired: 1 in]
            n164 = call "calibrate trap data V3RG.vi"("array of calibration clusters"=w341, "Trap position array"=w265, "MCL offset scanning range (V)"="MCL offset scanning range (V)", "Multi-MCL offset array"="Multi-MCL offset array", "two trap offset values"="Two Trap Offset Values", "Dynamic offset update"="Dynamic offset\nupdate", "Multiple-MCL offset?"="Multiple-MCL offset?", "x (true) or y (false)"=TRUE, "Data array"=w337, "Offset File step size"="Offset file step size") -> ("Positions out"=w338:dbl[][], "Forces out (pN)"=w339:dbl[][])
            n165 = Unbundle(w263) -> ("Output trap positions[0]"=w262:cluster{"X":dbl[], "Y":dbl[]}, "Output trap positions[1]"=w261:cluster{"X":dbl[], "Y":dbl[]}, "Output trap positions[2]"=w260:cluster{"X":dbl[], "Y":dbl[]})
            n166 = feedback #4(i16 0) -> (w218:i16)
            n167 = call "correlation scan.vi"("Correlations in"=w210, "Voltages in"=w207, "Cycle counter"=w218, "in put Array"=w201, "T3 positioning \ntest range (V)"="T3 positioning test range (V)", "Number of acquisition cycles"=w215, "Scanning?"=w214) -> ("Voltages out"=w206:cluster{"X":dbl, "Y":dbl}, "Scanning out"=w205:bool, "Output array"=w200:dbl[][], "Cycle counter out"=w217:i16)
            n168 = feedback-in #1(w200) -> ()
            n169 = feedback-in #4(w217) -> ()
            n170 = local read "Mean Trap Positions (nm)"() -> (w251:T5)
            n171 = local write "Correlation scanning"(w205) -> ()
            n172 = case shown="True" w205 {
              tunnel: w206 -> [_ w365]
              frame False {
              }
              frame True {
                n173 = Unbundle By Name(w365) -> ("X"=w364:dbl, "Y"=w363:dbl)
                n174 = local write "Trap 3 X (V)"(w364) -> ()
                n175 = local write "Trap 3 Y (V)"(w363) -> ()
              }
            }
            n176 = Build Array("Trap 1 Bead Size (nm)", "Trap 2 Bead Size (nm)", "Trap 3 Bead Size (nm)") -> (w237:dbl[])
            n177 = call "Force and position waveforms.vi"("Input waveforms"=w337, "Forces  (pN)"=w339, "Deflections (nm)"=w338, "Mean Trap Positions (nm)"="Mean Trap Positions (nm)") -> ("Absolute Positions"=w238:waveform(dbl)[], "Forces"=w231:waveform(dbl)[], "Deflections"=w278:waveform(dbl)[], "Raw Data"=w277:waveform(dbl)[])  [unwired: 1 out]
            n178 = Unbundle(w262) -> ("X"=w259:dbl[])  [unwired: 1 out]
            n179 = Unbundle(w261) -> ("X"=w258:dbl[])  [unwired: 1 out]
            n180 = Unbundle(w260) -> ("X"=w257:dbl[], "Y"=w256:dbl[])
            n181 = Unbundle By Name("T3 positioning test range (V)") -> ("Xmax"=w196:dbl, "Xmin"=w195:dbl, "increment"=w190:dbl, "Ymax"=w194:dbl, "Ymin"=w193:dbl)
            n182 = Index Array(array=w200, index (col)=3) -> (element=w198:dbl[])  [unwired: 1 in]
            n183 = Index Array(array=w200, index (col)=2) -> (element=w199:dbl[])  [unwired: 1 in]
            n184 = Subtract(x=w194, y=w193) -> (x-y=w191:dbl)
            n185 = Subtract(x=w196, y=w195) -> (x-y=w192:dbl)
            n186 = call "1D force plotting.vi"("Calibration"="Calibration", "Forces"=w231, "Deflections"=w278, "Raw Data"=w277) -> ("Output force values"=w331:T16, "Output waveforms"=→"Force":waveform(dbl)[])  [unwired: 1 in, 1 out]
            n187 = call "2D force plotting.vi"("Trap positions"=w264, "Calibration"="Calibration 2", "Bead sizes"=w237, "Raw Data"=w277, "Deflections"=w278, "Forces"=w231, "Absolute Positions"=w238) -> ("Output waveforms"=→"2D forces":waveform(dbl)[], "Output"=→"Force (pN)":T3, "Junctions"=w242:cluster{"X":dbl[], "Y":dbl[]}[], "deflection lines"=w243:cluster{"X":dbl[], "Y":dbl[]}[], "tether sizes"=w233:dbl[][])
            n188 = Index Array(array=w259, index=0) -> (element=w250:dbl)
            n189 = Index Array(array=w258, index=0) -> (element=w249:dbl)
            n190 = Index Array(array=w257, index=0) -> (element=w248:dbl)
            n191 = Index Array(array=w256, index=0) -> (element=w244:dbl)
            n192 = Quotient & Remainder(x=w191, y=w190) -> (floor(x/y)=w188:dbl)  [unwired: 1 out]
            n193 = Quotient & Remainder(x=w192, y=w190) -> (floor(x/y)=w189:dbl)  [unwired: 1 out]
            n194 = Increment(x=w189) -> (x+1=w186:dbl)
            n195 = Increment(x=w188) -> (x+1=w187:dbl)
            n196 = Bundle By Name(cluster=w251, "T1 X"=w250, "T2 X"=w249, "T3 X"=w248, "T3 Y"=w244) -> (w247:T5)
            n197 = Reshape Array(w198, w186, w187) -> (→"Intensity Graph Y":dbl[][])
            n198 = Reshape Array(w199, w186, w187) -> (→"Intensity Graph X":dbl[][])
            n199 = Unbundle By Name(w331) -> ("T1 X"=→"T1 X":dbl, "T2 X"=→"T2 X":dbl, "Mean"=→"Mean":dbl, "Difference"=→"Difference":dbl)
            n200 = local write "Mean Trap Positions (nm)"(w247) -> ()
            n201 = Build Array (concatenate)(w264, w243, w242) -> (→"Positions \nand displacements":cluster{"X":dbl[], "Y":dbl[]}[])
            n202 = call "2D tether waveforms.vi"("tether sizes"=w233, "Data period (s)"=w235, "Time Stamp"=w234, "Forces"=w231) -> ("tethers"=→"2D tethers":waveform(dbl)[], "output forces"=→"tether forces":waveform(dbl)[])  [unwired: 2 in, 1 out]
          }
        }
      }
    }
  }
